vi "Timed Loop Offset.vi"() -> ()   [LabVIEW 2023]
doc: "This example illustrates the role of the offset for a Timed Loop. Two loops, A and B, plot a spike at their expected start times, to illustrate when they started in relationship to each other."
uses:
  <vilib>/Platform/TimedLoop/XDataNode/timing_clust.ctl
  <vilib>/Platform/TimedLoop/XDataNode/nitl_modes.ctl
  <vilib>/Platform/TimedLoop/XDataNode/wakeup.ctl
  <vilib>/platform/TimedLoop/XDataNode/XDataNode.xnode
  <vilib>/Platform/TimedLoop/XDataNode/XDNodeRunTimeDep.lvlib
panel:
  out "Timed Loop Iteration Start Times":i64[][](graph)
  in  "Offset Loop B":i64=5
  in  "Offset Loop A":i64
  in  "Period Loop B":i64=10
  in  "Period Loop A":i64=10
  # "Overview: Demonstrates the significance of the Offset configuration value on a Timed Loop.\nRequirements: Windows\nInstructions:\nRun the VI. Observe the offset between the spikes in Loop A and Loop B. See the block diagram for more information."
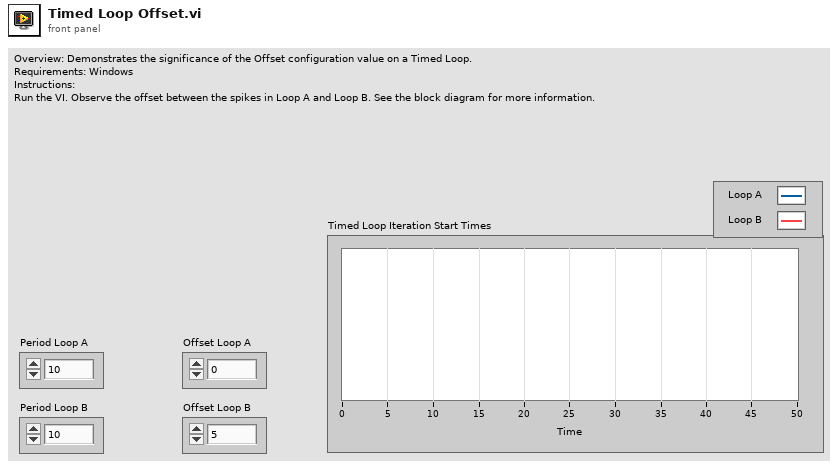
[diagram p1: front panel]
types:
  T1 = typedef "XDNodeRunTimeDep.lvlib/timing_clust.ctl" = cluster{"Expected End [f-1]":u64, "Actual End [f-1]":u64, "Finished Late? [f-1]":bool, "Expected End [i-1]":u64, "Actual End [i-1]":u64, "Finished Late? [i-1]":bool, "Expected Start [i]":u64, "Actual Start [i]":u64, "Expected Start [f]":u64, "Actual Start [f]":u64, "Source Name":string, "Structure Name":string, "Period":i64, "Deadline":i64, "Offset":i64, "Start":i64, "Priority":i32, "Timeout":i32, "Mode":T2, "Wakeup Reason":T3, "Error":errorcluster, "Source Type":string, "Secondary Source Type":string, "Global End Time":u64, "Global Start Time":u64, "Frame Duration":u64, "Iteration Duration":u64, "Assigned CPU":i32, "I/O Scan Engine Mode":u32}
  T2 = typedef "XDNodeRunTimeDep.lvlib/nitl_modes.ctl" = enum32{"No Change", "Process missed periods, maintain original phase", "Discard missed periods, maintain original phase", "Process missed periods, ignore original phase", "Discard missed periods, ignore original phase"}
  T3 = typedef "XDNodeRunTimeDep.lvlib/wakeup.ctl" = enum32{"Normal", "Aborted", "Asynchronous wakeup", "Timing source error", "Timed loop error", "Timeout"}
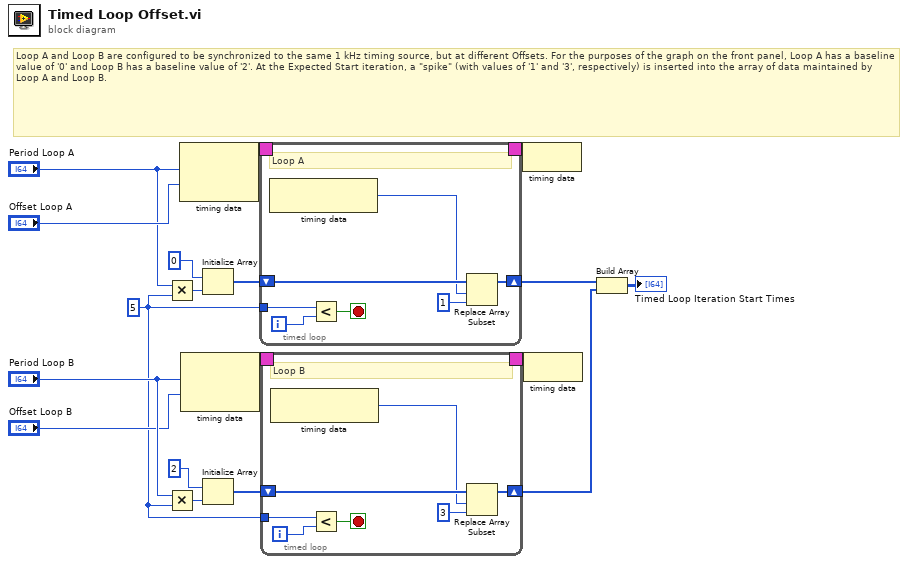
[diagram p0: block diagram]
diagram:
  w10 = i64 5
  # "Loop A and Loop B are configured to be synchronized to the same 1 kHz timing source, but at different Offsets. For the purposes of the graph on the front panel, Loop A has a baseline value of '0' and Loop B has a baseline value of '2'. At the Expected Start iteration, a \"spike\" (with values of '1' and '3', respectively) is inserted into the array of data maintained by Loop A and Loop B."
  n1 = Multiply(x="Period Loop A", y=w10) -> (x*y=w9:i64)
  n2 = Multiply(x="Period Loop B", y=w10) -> (x*y=w6:i64)
  n3 = node-c288("Period Loop A", "Offset Loop A") -> (w16:T1)
  n4 = node-c288("Period Loop B", "Offset Loop B") -> (w18:T1)
  n5 = Initialize Array(i64 0, w9) -> (w8:i64[])
  n6 = Initialize Array(i64 2, w6) -> (w5:i64[])
  n7 = timed-loop {
    shift-left: w8 -> [w22]
    shift-right: [w20] -> w2
    tunnel: w10 -> [w23]
    timing-out: [_] -> w15
    timing: w16 -> [_]
    i -> [w25]
    stop <- w24 stop-if-true
    # "Loop A"
    n8 = node-c288() -> (w19:i64)  [unwired: 1 in]
    n9 = Less?(x=w23, y=w25) -> (x < y?=w24:bool)
    n10 = Replace Array Subset(array=w22, new element=i64 1 ("new element/subarray"), index=w19) -> (w20:i64[])
  }
  n11 = timed-loop {
    shift-left: w5 -> [w32]
    shift-right: [w30] -> w1
    tunnel: w10 -> [w33]
    timing-out: [_] -> w17
    timing: w18 -> [_]
    i -> [w35]
    stop <- w34 stop-if-true
    # "Loop B"
    n12 = node-c288() -> (w29:i64)  [unwired: 1 in]
    n13 = Less?(x=w33, y=w35) -> (x < y?=w34:bool)
    n14 = Replace Array Subset(array=w32, new element=i64 3 ("new element/subarray"), index=w29) -> (w30:i64[])
  }
  n15 = node-c288(w15) -> ()
  n16 = node-c288(w17) -> ()
  n17 = Build Array(w2, w1) -> (→"Timed Loop Iteration Start Times":i64[][])
